vi "WT210 Check Harmonic Content.vi"(8 "error in (no error)":errorcluster, 11 "VISA Refnum in":refnum<visa-resource-name>) -> (0 "error out":errorcluster, 2 "VTHD":sgl format="%.3g", 3 "VISA Refnum out":refnum<visa-resource-name>)   [LabVIEW 2018]
uses:
  Yokogawa WT200 Series.lvlib
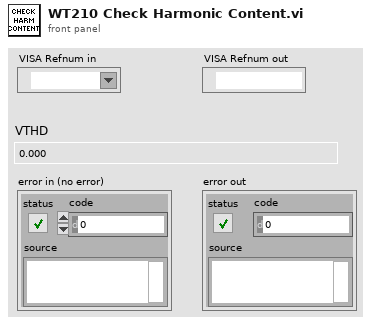
[diagram p1: front panel]
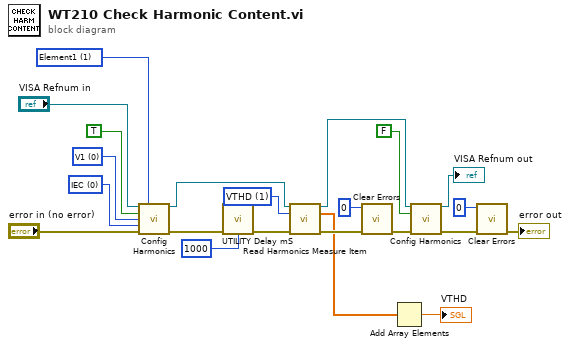
[diagram p0: block diagram]
diagram:
  w13 = u16 1 items=["Sync", "VTHD", "V", "VCON", "ATHD", "A", "ACON", "PF", "W", "WCON", "Vdeg", "Adeg"] ("Harmonics Item (2: V)")
  w7 = u16 0 items=["IEC", "CSA"] ("THD (0: IEC)")
  w6 = u16 0 items=["V1", "A1", "V2", "A2", "V3", "A3"] ("PLL source (0: V1)")
  w5 = u16 1 items=["", "Element1", "Element2", "Element3"] ("Element (1: Element 1)")
  n1 = call "Config Harmonics.vi"("VISA resource name"="VISA Refnum in", "Element (1: Element 1)"=w5, "Harmonic Mode (F: OFF)"=TRUE, "PLL source (0: V1)"=w6, "THD (0: IEC)"=w7, "error in (no error)"="error in (no error)") -> ("VISA resource name out"=w3:refnum<visa-resource-name>, "error out"=w10:errorcluster)  [unwired: 8 in]
  n2 = call "UTILITY Delay mS.vi"("Error In"=w10, "milliseconds to wait"=u32 1000) -> ("Error Out"=w16:errorcluster)  [unwired: 13 in]
  n3 = call "Read Harmonics Measure Item.vi"("VISA resource name"=w3, "Harmonics Item (2: V)"=w13, "error in (no error)"=w16) -> ("VISA resource name out"=w14:refnum<visa-resource-name>, "Data"=w2:sgl[], "error out"=w18:errorcluster)  [unwired: 10 in]
  n4 = call <vilib>:"Clear Errors.vi"("error in (no error)"=w18, "specific error code to clear (0: all)"=0) -> ("error out"=w19:errorcluster)  [unwired: 4 in, 1 out]
  n5 = Add Array Elements(numeric array=w2) -> (sum=→"VTHD":sgl)
  n6 = call "Config Harmonics.vi"("VISA resource name"=w14, "Harmonic Mode (F: OFF)"=FALSE, "error in (no error)"=w19) -> ("VISA resource name out"=→"VISA Refnum out":refnum<visa-resource-name>, "error out"=w21:errorcluster)  [unwired: 11 in]
  n7 = call <vilib>:"Clear Errors.vi"("error in (no error)"=w21, "specific error code to clear (0: all)"=0) -> ("error out"=→"error out":errorcluster)  [unwired: 4 in, 1 out]
